vi "ACTUALIZAR GRAFICA.vi"(8 "error in (no error)":errorcluster, 10 "event data":waveform(dbl), 11 "SEÑAL_ACTUALIZABLE in":refnum<class "  SEÑAL_ACTUALIZABLE.lvclass">) -> (0 "error out":errorcluster, 3 "SEÑAL_ACTUALIZABLE out":refnum<class "  SEÑAL_ACTUALIZABLE.lvclass">)   [LabVIEW 2019, in "  SEÑAL_ACTUALIZABLE.lvlib" / "  SEÑAL_ACTUALIZABLE.lvclass"]
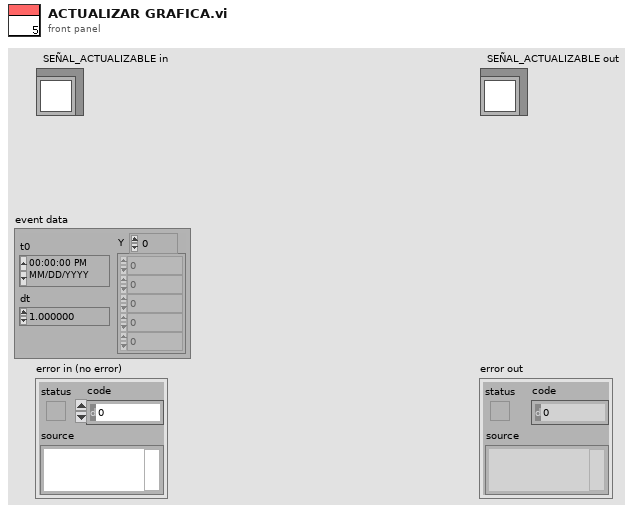
[diagram p1: front panel]
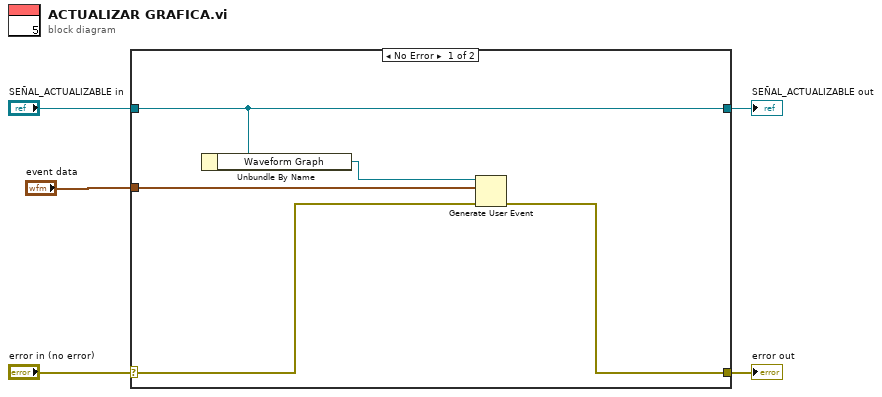
[diagram p0: block diagram]
diagram:
  n1 = case shown="No Error" "error in (no error)" {
    selector: "error in (no error)" -> [w7 w12]
    tunnel: [w6 w12] -> w4
    tunnel: [w10 w11] -> w2
    tunnel: "SEÑAL_ACTUALIZABLE in" -> [w10 w11]
    tunnel: "event data" -> [w8 _]
    frame No Error {
      n2 = Unbundle By Name(w10) -> ("Waveform Graph"=w9:refnum<user-event>)
      n3 = Generate User Event(user event=w9, event data cluster=w8, error in=w7) -> (error out=w6:errorcluster)  [unwired: 1 in, 1 out]
    }
    frame Error {
    }
  }
  "error out" <- w4
  "SEÑAL_ACTUALIZABLE out" <- w2
